vi "xhochy.vi"(8 "Base":dbl format="%#_13g", 11 "Exponent":i32) -> (0 "result":dbl)   [LabVIEW 2013]
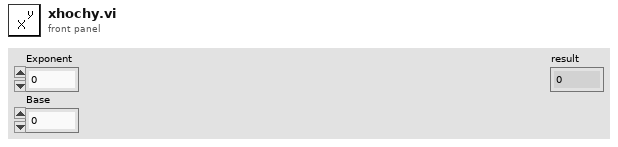
[diagram p1: front panel]
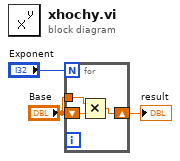
[diagram p0: block diagram]
diagram:
  n1 = for {
    N: "Exponent" -> [_]
    shift-right: [w6] -> w1
    shift-left: "Base" -> [w5]
    tunnel: "Base" -> [w4]
    n2 = Multiply(x=w4, y=w5) -> (x*y=w6:dbl)
  }
  "result" <- w1
